vi "Update Worktable Positions.vi"(8 "error in":errorcluster, 11 "Potting Procedure in":refnum<class "Potting Procedure.lvclass">) -> (0 "error out":errorcluster, 3 "Potting Procedure out":refnum<class "Potting Procedure.lvclass">)   [LabVIEW 2011, in "Potting Procedure.lvclass"]
uses:
  Potting Procedure.lvclass
  Shared Components/Gantry Class/Gantry Class.lvclass
  Shared Components/WorkTable Class/WorkTable Class.lvclass
  Shared Components/Vec3d Class/Vec3d Class.lvclass
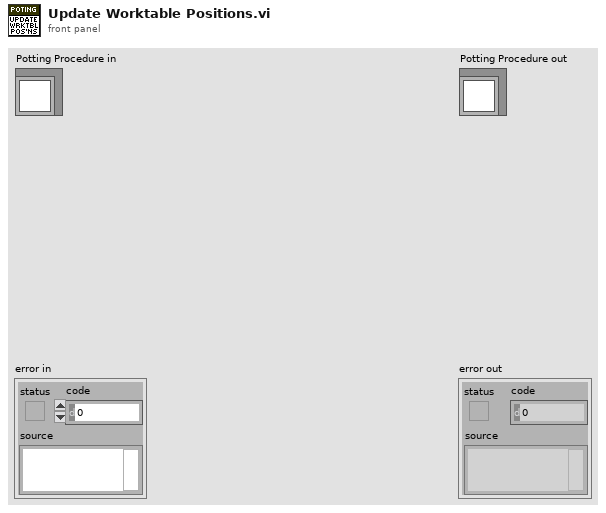
[diagram p1: front panel]
types:
  T1 = enum16{"Empty", "Unglued", "Stamped", "PartOnTop", "Weighted", "Unpotted", "Potted"}
  T2 = cluster{"Feature Coordinates":refnum<class "Vec3d Class.lvclass">, "Feature Name":string}
  T3 = typedef "Inspect Fiducials.ctl" = cluster{"Has Been Run?":bool, "Module-Chuck Fiducials":cluster{"Fiducials-HDI":T4[], "Fiducials-BBM":T4[], "Chuck":i32, "Slot":i32}[]}
  T4 = typedef "Fiducial Image.ctl" = cluster{"Fiducial Image":T5, "Selected Fiducial":T7, "fiducial name":string}
  T5 = typedef "Physical Image.ctl" = cluster{"Image Position":refnum<class "Vec3d Class.lvclass">, "Image Reference":T6, "Field of View":cluster{"x(mm)":dbl, "y(mm)":dbl}}
  T6 = typedef "IMAQ Image.ctl" = refnum<image>
  T7 = typedef "Fiducial with Source.ctl" = cluster{"Fiducial Image Coordinate":refnum<class "Vec3d Class.lvclass">, "Fiducial Source":enum16{"Pattern Recognition", "User", "Error", "Default"}}
  T8 = cluster{"Fiducials-HDI":T4[], "Fiducials-BBM":T4[], "Chuck":i32, "Slot":i32}[]
  T9 = cluster{"Feature Coordinates":refnum<class "Vec3d Class.lvclass">, "Feature Name":string}[]
  T10 = typedef "Position_Orientation.ctl" = cluster{"Center":refnum<class "Vec3d Class.lvclass">, "Orientation":refnum<class "Orient3d Class.lvclass">}
  T11 = typedef "Worktable_Module Slot.ctl" = cluster{"Slot State":enum16{"Empty", "Unglued", "Stamped", "PartOnTop", "Weighted", "Unpotted", "Potted"}, "BBM Type":enum16{"None", "BBM", "GlassSlide"}, "HDI Type":enum16{"None", "HDI", "Polyimide"}, "Vacuum Channel":u8, "Location/Orientation BBM":T10, "Location/Orientation HDI":T10, "S/N":string}
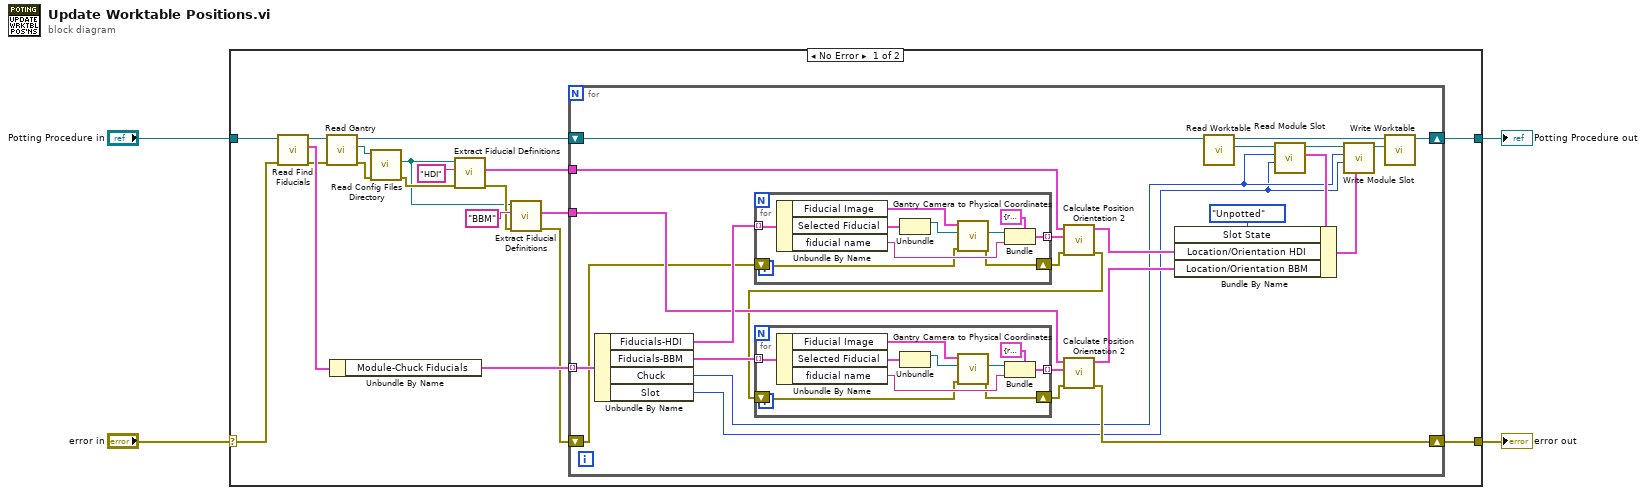
[diagram p0: block diagram]
diagram:
  n1 = case shown="No Error" "error in" {
    selector: "error in" -> [w12 w70]
    tunnel: [w5 w70] -> w3
    tunnel: [w13 w69] -> w1
    tunnel: "Potting Procedure in" -> [w23 w69]
    frame No Error {
      n2 = call-dynamic "Read Find Fiducials.vi"("error in (no error)"=w12, "Potting Procedure in"=w23) -> ("error out"=w11:errorcluster, "Find Fiducials"=w22:T3, "Potting Procedure out"=w10:refnum<class "Potting Procedure.lvclass">)  [unwired: 7 in]
      n3 = call-dynamic "Read Gantry.vi"("error in (no error)"=w11, "Potting Procedure in"=w10) -> ("error out"=w9:errorcluster, "Gantry"=w20:refnum<class "Gantry Class.lvclass">, "Potting Procedure out"=w14:refnum<class "Potting Procedure.lvclass">)  [unwired: 7 in]
      n4 = Unbundle By Name(w22) -> ("Module-Chuck Fiducials"=w21:T8)
      n5 = call-dynamic "Read Config Files Directory.vi"("error in (no error)"=w9, "Gantry Class in"=w20) -> ("error out"=w8:errorcluster, "Config Files Directory"=w6:path)  [unwired: 7 in, 1 out]
      n6 = call "Extract Fiducial Definitions.vi"("error in"=w8, "Part Name"="HDI", "Config Location"=w6) -> ("error out"=w17:errorcluster, "Feature Definitions"=w15:T9)  [unwired: 7 in]
      n7 = call "Extract Fiducial Definitions.vi"("error in"=w17, "Part Name"="BBM", "Config Location"=w6) -> ("error out"=w7:errorcluster, "Feature Definitions"=w16:T9)  [unwired: 7 in]
      n8 = for {
        tunnel: w21 -> [w48] mode=indexing
        tunnel: w16 -> [w44]
        tunnel: w15 -> [w46]
        shift-right: [w33] -> w13
        shift-left: w14 -> [w36]
        shift-right: [w37] -> w5
        shift-left: w7 -> [w43]
        n9 = Unbundle By Name(w48) -> ("Fiducials-HDI"=w47:T4[], "Fiducials-BBM"=w41:T4[], "Chuck"=w25:i32, "Slot"=w24:i32)
        n10 = for {
          tunnel: w47 -> [w68] mode=indexing
          tunnel: [w61] -> w45 mode=indexing
          shift-right: [w59] -> w42
          shift-left: w43 -> [w60]
          n11 = Unbundle By Name(w68) -> ("Fiducial Image"=w66:T5, "Selected Fiducial"=w67:T7, "fiducial name"=w62:string)
          n12 = Unbundle(w67) -> ("Fiducial Image Coordinate"=w65:refnum<class "Vec3d Class.lvclass">)  [unwired: 1 out]
          n13 = call "Gantry Camera to Physical Coordinates.vi"("error in"=w60, "Image Coordinate"=w65, "Physical Image"=w66) -> ("error out"=w59:errorcluster, "Global Coordinate"=w63:refnum<class "Vec3d Class.lvclass">)  [unwired: 6 in, 1 out]
          n14 = Bundle(cluster=T2 {"Feature Coordinates"=refnum, "Feature Name"=""} ("Feature Description"), "Feature Coordinates"=w63, "Feature Name"=w62) -> (w61:T2)
        }
        n15 = call "Calculate Position Orientation 2.vi"("error in"=w42, "Measured Global Positions"=w45, "Known Local Positions"=w46) -> ("error out"=w39:errorcluster, "PositionOrientation"=w28:T10)  [unwired: 6 in, 1 out]
        n16 = for {
          tunnel: w41 -> [w58] mode=indexing
          tunnel: [w51] -> w40 mode=indexing
          shift-right: [w49] -> w38
          shift-left: w39 -> [w50]
          n17 = Unbundle By Name(w58) -> ("Fiducial Image"=w56:T5, "Selected Fiducial"=w57:T7, "fiducial name"=w52:string)
          n18 = Unbundle(w57) -> ("Fiducial Image Coordinate"=w55:refnum<class "Vec3d Class.lvclass">)  [unwired: 1 out]
          n19 = call "Gantry Camera to Physical Coordinates.vi"("error in"=w50, "Image Coordinate"=w55, "Physical Image"=w56) -> ("error out"=w49:errorcluster, "Global Coordinate"=w53:refnum<class "Vec3d Class.lvclass">)  [unwired: 6 in, 1 out]
          n20 = Bundle(cluster=T2 {"Feature Coordinates"=refnum, "Feature Name"=""} ("Feature Description"), "Feature Coordinates"=w53, "Feature Name"=w52) -> (w51:T2)
        }
        n21 = call "Calculate Position Orientation 2.vi"("error in"=w38, "Measured Global Positions"=w40, "Known Local Positions"=w44) -> ("error out"=w37:errorcluster, "PositionOrientation"=w27:T10)  [unwired: 6 in, 1 out]
        n22 = call-dynamic "Read Worktable.vi"("Potting Procedure in"=w36) -> ("WorkTable out"=w31:refnum<class "WorkTable Class.lvclass">, "Potting Procedure out"=w35:refnum<class "Potting Procedure.lvclass">)  [unwired: 8 in, 1 out]
        n23 = call-dynamic "Read Module Slot.vi"("slot"=w24, "chuck"=w25, "WorkTable in"=w31) -> ("Module Slot"=w29:T11, "WorkTable out"=w30:refnum<class "WorkTable Class.lvclass">)  [unwired: 6 in, 1 out]
        n24 = Bundle By Name(cluster=w29, "Slot State"=T1."Unpotted", "Location/Orientation HDI"=w28, "Location/Orientation BBM"=w27) -> (w32:T11)
        n25 = call-dynamic "Write Module Slot.vi"("Module Slot"=w32, "slot"=w24, "chuck"=w25, "WorkTable in"=w30) -> ("WorkTable out"=w34:refnum<class "WorkTable Class.lvclass">)  [unwired: 6 in, 1 out]
        n26 = call-dynamic "Write Worktable.vi"("WorkTable in"=w34, "Potting Procedure in"=w35) -> ("Potting Procedure out"=w33:refnum<class "Potting Procedure.lvclass">)  [unwired: 8 in, 1 out]
      }
    }
    frame Error {
    }
  }
  "error out" <- w3
  "Potting Procedure out" <- w1
